vi "MDF4 Close Stream.vi"(8 "Error In":errorcluster, 11 "Stream Reference in":i64) -> (0 "Error Out":errorcluster, 3 "Stream Reference out":i64)   [LabVIEW 2019, in "MD4Logger Engine.lvlib"]
uses:
  MD4Logger Engine.lvlib
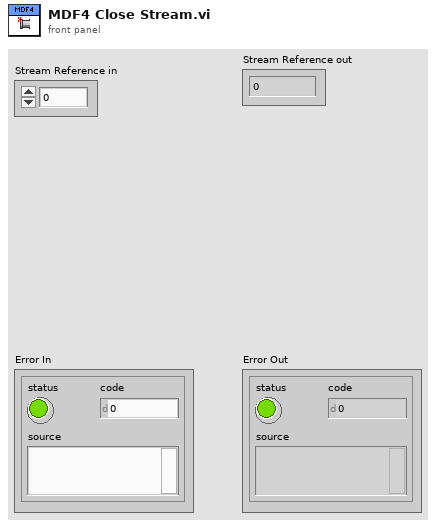
[diagram p1: front panel]
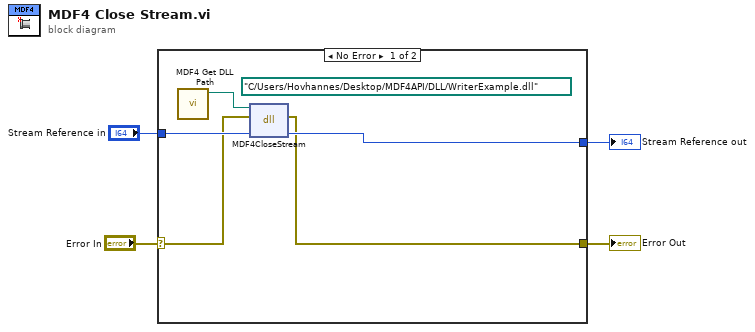
[diagram p0: block diagram]
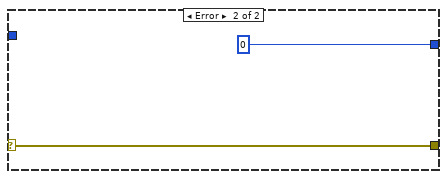
[diagram p2: hidden frame]
diagram:
  n1 = case shown="No Error" "Error In" {
    selector: "Error In" -> [w8 w11]
    tunnel: "Stream Reference in" -> [w9 _]
    tunnel: [w6 w11] -> w2
    tunnel: [w7 i64 0 ("m4")] -> w1
    frame No Error {
      (unwired) path "C:/Users/Hovhannes/Desktop/MDF4API/DLL/WriterExample.dll" ("path in")
      n2 = call "MDF4 Get DLL Path.vi"() -> ("DLL Path Out"=w5:path)  [unwired: 11 in]
      n3 = dll-call lib="C:/Users/Hovhannes/Desktop/MDF4API/DLL/WriterExample.dll" fn="MDF4CloseStream"(path in=w5, error in=w8, "DStream"=w9) -> (error out=w6:errorcluster, "DStream"=w7:i64)  [unwired: 2 in, 1 out]
    }
    frame Error {
    }
  }
  "Error Out" <- w2
  "Stream Reference out" <- w1
